vi "Begin-End Array.vi"(8 "Error In":errorcluster) -> (0 "Error Out":errorcluster)   [LabVIEW 2017, in "Tests.lvlib" / "Writer.lvlib"]
uses:
  Writer.lvlib
  src/LabPack/Public/Writer/Private/Begin by Value.vi
  src/LabPack/Public/Writer/Private/Begin Array by Value.vi
  src/LabPack/Public/Writer/Private/End Array by Value.vi
  src/LabPack/Public/Writer/Private/End by Value.vi
  src/LabPack/Public/Writer/Writer.lvclass
  <vilib>/addons/_JKI Toolkits/Caraya/classes/Test/Test.lvclass
  <vilib>/addons/_JKI Toolkits/Caraya/classes/Assert/Assert.lvclass
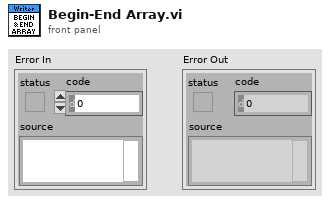
[diagram p1: front panel]
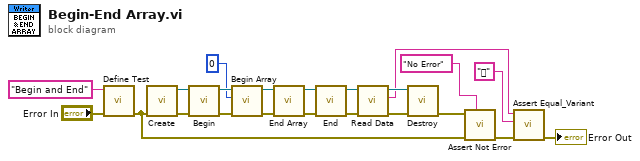
[diagram p0: block diagram]
diagram:
  n1 = call <vilib>:"Define Test.vi"("error in (no error)"="Error In", "Label (VI Title)"="Begin and End") -> ("error out"=w17:errorcluster)  [unwired: 9 in]
  n2 = call "Create.vi"("Error In"=w17) -> ("Error Out"=w15:errorcluster, "Writer"=w18:refnum<class "Writer.lvclass">)  [unwired: 9 in]
  n3 = call-poly "Begin.vi"("Error In"=w15, "Writer In"=w18) -> ("Error Out"=w11:errorcluster, "Writer Out"=w13:refnum<class "Writer.lvclass">)  [unwired: 8 in]
  n4 = call-poly "Begin Array.vi"("Error In"=w11, "Elements Count"=u32 0, "Writer In"=w13) -> ("Error Out"=w8:errorcluster, "Writer Out"=w12:refnum<class "Writer.lvclass">)  [unwired: 7 in]
  n5 = call-poly "End Array.vi"("Error In"=w8, "Writer In"=w12) -> ("Error Out"=w7:errorcluster, "Writer Out"=w9:refnum<class "Writer.lvclass">)  [unwired: 8 in]
  n6 = call-poly "End.vi"("Error In"=w7, "Writer In"=w9) -> ("Error Out"=w5:errorcluster, "Writer Out"=w14:refnum<class "Writer.lvclass">)  [unwired: 8 in]
  n7 = call "Read Data.vi"("Error In"=w5, "Writer In"=w14) -> ("Error Out"=w4:errorcluster, "Data"=w2:string, "Writer Out"=w6:refnum<class "Writer.lvclass">)  [unwired: 7 in]
  n8 = call "Destroy.vi"("Error In"=w4, "Writer"=w6) -> ("Error Out"=w16:errorcluster)  [unwired: 9 in]
  n9 = call <vilib>:"Assert Not Error.vi"("Label"="No Error", "error in (no error)"=w17, "Not Error?"=w16) -> ("error out"=w20:errorcluster)  [unwired: 8 in]
  n10 = call <vilib>:"Assert Equal_Variant.vi"("error in (no error)"=w20, "Y"="" ("Data"), "X"=w2) -> ("error out"=→"Error Out":errorcluster)  [unwired: 8 in]
